vi "例程46-条件结构巧用.vi"() -> ()   [LabVIEW 2016]
panel:
  out "字符串":string
  in  "按钮3":bool
  in  "按钮2":bool
  in  "按钮1":bool
  in  "停止":bool
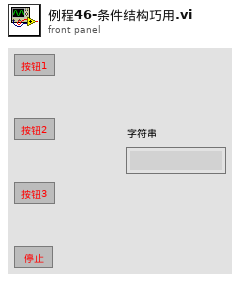
[diagram p1: front panel]
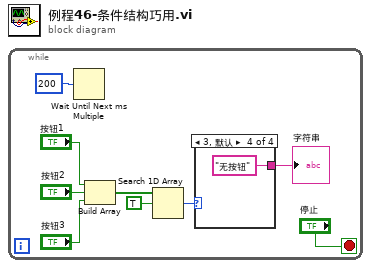
[diagram p0: block diagram]
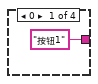
[diagram p2: hidden frame]
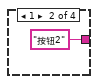
[diagram p3: hidden frame]
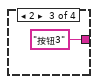
[diagram p4: hidden frame]
diagram:
  n1 = while {
    stop <- "停止" stop-if-true
    n2 = Wait Until Next ms Multiple(millisecond multiple=u32 200 ("毫秒倍数")) -> ()  [unwired: 1 out]
    n3 = Build Array("按钮1", "按钮2", "按钮3") -> (w5:bool[])
    n4 = Search 1D Array(1D array=w5, element=TRUE ("元素")) -> (index of element=w2:i32)  [unwired: 1 in]
    n5 = case shown="3, 默认" w2 {
      tunnel: ["按钮1" "按钮2" "按钮3" "无按钮"] -> w3
      frame 0 {
      }
      frame 1 {
      }
      frame 2 {
      }
      frame 3, Default {
      }
    }
    "字符串" <- w3
  }
